vi "Calculate Baseline.vi"(0 "widthOfSequence":i32, 4 "threshold":u16, 6 "minPointsInBaseline":i32, 7 "error in (no error)":errorcluster, 8 "size":i32, 9 "array":u16[](array[numeric]), 10 "endInitBaseline":i32, 11 "startInitBaseline":i32) -> (1 "Stdev":i16, 2 "Baseline":i16, 3 "error out":errorcluster)   [LabVIEW 2013]
doc: "<B>Explanation of params</B>\nA description is included at the bottom.\n<B>int32_t findBaseline</B>: The return value for the function, a 0 (zero) means a baseline is found\n a value >= 5000 indicates the occurrence of an error.\n<B>int32_t startInitBaseline</B>: The initial starting value for calculating the baseline, in most cases \n this value should be 0 (zero). \n<B>int32_t endInitBaseline</B>: The initial maximum element that is included in the baseline. If a\n pulse occurres before this element the calculation stops there.\n<B>uint16_t array[]</B>: The array which holds the event data.\n<B>const int32_t size</B>: The size of the event data array.\n<B>const uint16_t threshold</B>: This value determines if an element is part of the baseline or\n belongs to a pulse.\n<B>const int32_t widthOfSequence</B>: If the number of elements in the initial baseline is less\n than <B>minPointsInBaseline</B> a new starting value for calculating the\n baseline is determined by using two sequences i.e. subarrays of width\n <B>widthOfSequence</B>.\n<B>int32_t minPointsInBaseline</B>: Defines the minimal number of elements that should be\n present in the baseline.\n <B>int16_t *Baseline</B>: A pointer to the calculated baseline. LABVIEW handles this as a\n pointer to value, so this value holds the baseline.\n<B>int16_t *Stdev</B>: A pointer to the calculated standard deviation. LABVIEW handles this as a\n pointer to value, so this value holds the standard deviation.\n\n<B>Description</B> \nThis Vi finds the baseline and corresponding standard deviation, providing an event data array with a supplied size. The initial baseline is calculated from <B>startInitBaseline</B> to <B>endInitBaseline</B>, by using the <B>threshold</B> to determine when an element is no longer part of the baseline. If the calculation stops before <B>minPointsInBaseline</B> is reached, the new <B>startInitBaseline</B> is determined using two sequences i.e. subarrays of width <B>widthOFSequence</B>. Both sequences are compared and if the next sequence is less smooth than the current sequence the start of the current sequence is picked as the new starting point for calculating the baseline. In the end the baseline and standard deviation are returned. If no baseline can be found both the <B>Baseline</B> and the <B>Stdev</B> get a value of <B>-999</B>"
uses:
  project/Baseline/Release/Baseline.dll
  <userlib>/Baseline/Baseline.lvlib
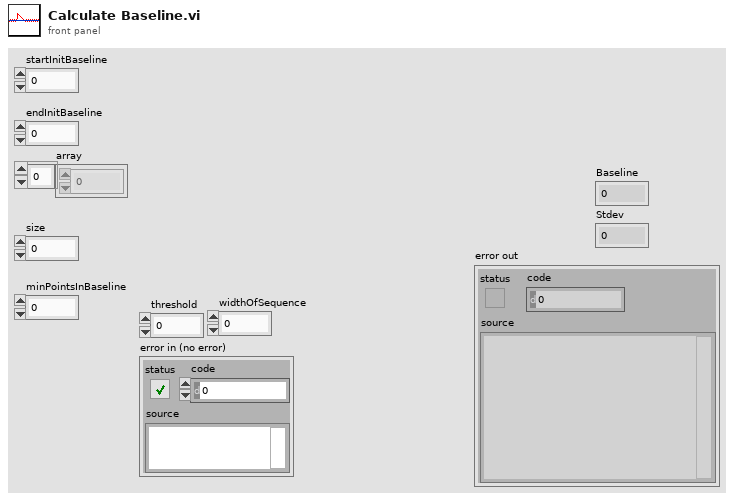
[diagram p1: front panel]
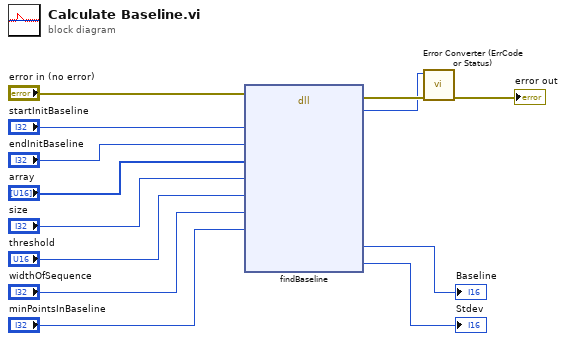
[diagram p0: block diagram]
diagram:
  n1 = dll-call lib="C:/Users/SuperUser/Documents/HiSparc/HISPARC_baseline/project/Baseline/Release/Baseline.dll" fn="findBaseline"(error in="error in (no error)", "startInitBaseline"="startInitBaseline", "endInitBaseline"="endInitBaseline", "array"="array", "size"="size", "threshold"="threshold", "widthOfSequence"="widthOfSequence", "minPointsInBaseline"="minPointsInBaseline") -> (error out=w6:errorcluster, "errorValue"=w5:i32, "Baseline"=→"Baseline":i16, "Stdev"=→"Stdev":i16)  [unwired: 11 in, 1 out]
  n2 = call "Error Converter (ErrCode or Status).vi"("error in (no error)"=w6, "error code"=w5) -> ("error out"=→"error out":errorcluster)  [unwired: 9 in]
